vi "Parse SSH_FXP_HANDLE.vi"(8 "error in":errorcluster, 11 "payload":u8[](array[numeric])) -> (0 "error out":errorcluster, 3 "handle":T1 format="%02x")   [LabVIEW 2020, in "NI_SFTP.lvlib"]
uses:
  <vilib>/net/SFTP/NI_SFTP.lvlib
  <vilib>/net/SFTP/Session/Handle.ctl
  fe9cab8e-2cf0-3fe7-1c9b-f8983c6ade3f.vi
  <vilib>/Bit Manipulation/Network-Order Bytes To Words Poly.vi
  <vilib>/Bit Manipulation/wrappers/Network-Order Bytes To Words/Network-Order Bytes To Words U32.vi
  <vilib>/net/SFTP/Low Level Connection/Low Level Connection.lvclass
  <vilib>/net/SFTP/Session/Session.lvclass
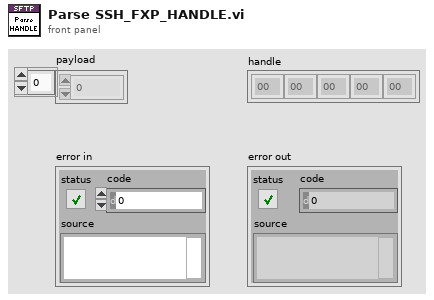
[diagram p1: front panel]
types:
  T1 = typedef "NI_SFTP.lvlib/Session.lvclass/Handle.ctl" = u8[]
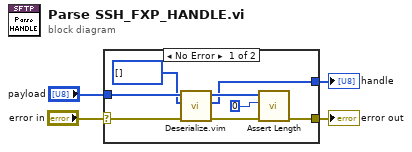
[diagram p0: block diagram]
diagram:
  n1 = case shown="No Error" "error in" {
    selector: "error in" -> [w11 w13]
    tunnel: [w7 w13] -> w3
    tunnel: "payload" -> [w12 _]
    tunnel: [w5 _] -> w1
    frame No Error {
      n2 = call "Deserialize.vim"("error in"=w11, "type"=T1 [], "bytes"=w12) -> ("error out"=w8:errorcluster, "value"=w5:u8[], "remaining bytes"=w9:u8[])  [unwired: 6 in]
      n3 = call <vilib>:"Assert Length.vi"("error in"=w8, "asserted length"=u32 0, "string in"=w9) -> ("error out"=w7:errorcluster)  [unwired: 7 in, 1 out]
    }
    frame Error {
    }
  }
  "error out" <- w3
  "handle" <- w1
